vi "Test Turning Point.vi"() -> ()   [LabVIEW 2014]
uses:
  ZScan.ctl
panel:
  out "Z @ Max Sharpness":dbl
  out "Max Sharpness":sgl
  out "Waveform Chart":dbl(graph)
  out "XY Graph":cluster{"Displacements":dbl[], dbl[]}[](graph)
  in  "Focus Parameters":T1={"Z0"=3.0, "f0"=100.0, "curvature"=3.0, "noise"=2.0}
  in  "Z Scan Parameters":T2={"Z Range"=20.0, "Resolution"=1.0, "Initial Direction"=enum."Up", "Focus Threshold"=970.0, "Ascent Constant"=0.1} {"Focus Threshold" min=0.0 max=1000.0 step=1.0 format="%#_2f"; "Ascent Constant" min=0.0 max=1000.0 step=1.0 format="%#_2f"; "Resolution" min=0.0 max=1.0 step=0.01 format="%_2g"; "Z Range" format="%_3g"}
  # "LICENSED MATERIALS – PROPERTY OF IBM\nCopyright IBM Corp. 2016,\nALL RIGHTS RESERVED"
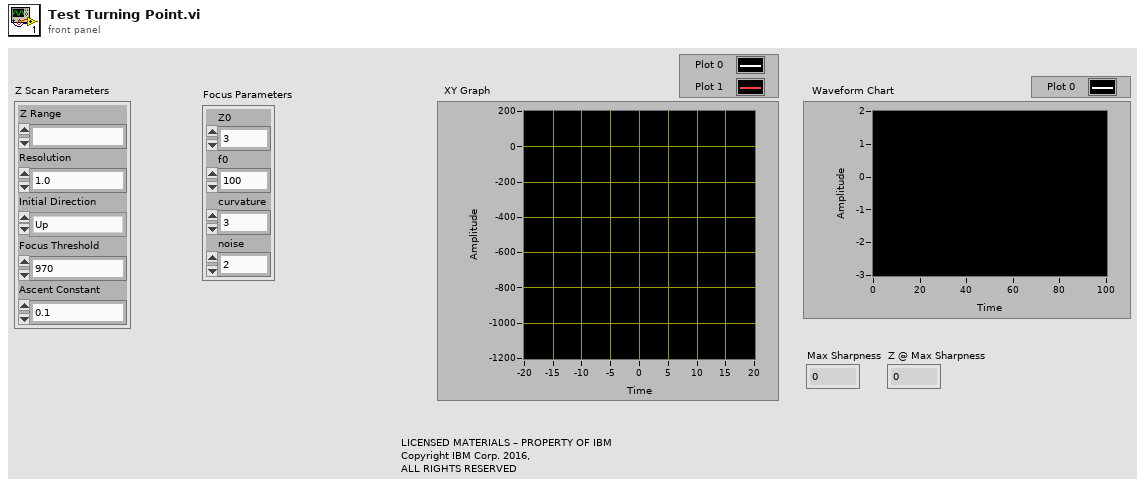
[diagram p1: front panel]
types:
  T1 = cluster{"Z0":dbl, "f0":dbl, "curvature":dbl, "noise":dbl}
  T2 = typedef "ZScan.ctl" = cluster{"Z Range":ext, "Resolution":dbl, "Initial Direction":enum16{"Up", "Down"}, "Focus Threshold":dbl, "Ascent Constant":dbl}
  T3 = cluster{"Registers Filled?":bool, "Negative Edge Slope?":bool, "Negative Z Slope?":bool, "Focus at Edge?":bool}
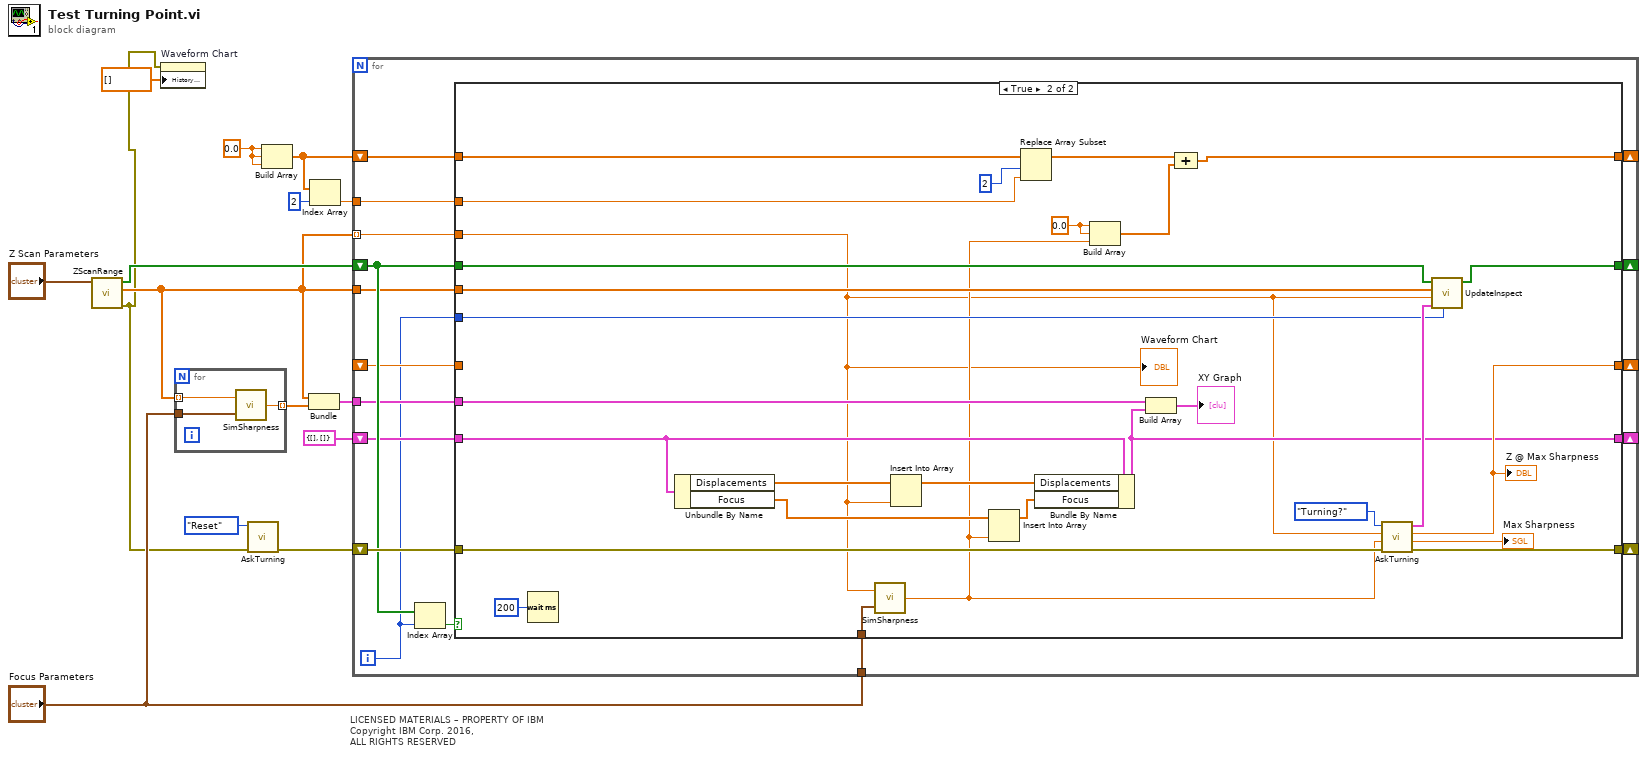
[diagram p0: block diagram]
diagram:
  w13 = 0.0 ("element")
  # "LICENSED MATERIALS – PROPERTY OF IBM\nCopyright IBM Corp. 2016,\nALL RIGHTS RESERVED"
  n1 = call "ZScanRange.vi"("Z Scan Parameters"="Z Scan Parameters") -> ("error out"=w1:errorcluster, "Displacements"=w5:dbl[], "Inspect?"=w8:bool[])  [unwired: 8 in]
  n2 = property on="Waveform Chart" class="WFChart (strict)"(error in=w1, "History Data"=dbl[] []) -> ()  [unwired: 1 in, 2 out]
  n3 = for {
    tunnel: "Focus Parameters" -> [w18]
    tunnel: [w17] -> w6 mode=indexing
    tunnel: w5 -> [w16] mode=indexing
    n4 = call "SimSharpness.vi"("Focus Parameters"=w18, "Z"=w16) -> ("Sharpness"=w17:dbl)
  }
  n5 = call "AskTurning.vi"("error in (no error)"=w1, "Function"=enum16{"Turning?", "Reset"}."Reset") -> ("error out"=w14:errorcluster)  [unwired: 6 in, 3 out]
  n6 = Build Array(w13, w13, w13) -> (w11:dbl[])
  n7 = Bundle("Displacements"=w5, w6) -> (w4:cluster{"Displacements":dbl[], dbl[]})  [unwired: 1 in]
  n8 = Index Array(array=w11, index=2) -> (element=w10:dbl)
  n9 = for {
    shift-right: [w33] -> _
    shift-left: w14 -> [w35]
    shift-right: [w32] -> _
    shift-left: w11 -> [w34]
    shift-right: [w31] -> _
    shift-left: w8 -> [w29]
    tunnel: w5 -> [w28]
    shift-right: [w27] -> _
    shift-left: _ -> [w26]
    tunnel: w5 -> [w24] mode=indexing
    tunnel: w10 -> [w25]
    tunnel: "Focus Parameters" -> [w23]
    tunnel: w4 -> [w22]
    shift-right: [w20] -> _
    shift-left: cluster{"Displacements":dbl[], "Focus":dbl[]} {"Displacements"=[], "Focus"=[]} -> [w21]
    i -> [w19]
    n10 = Index Array(array=w29, index=w19) -> (element=w30:bool)
    n11 = case shown="True" w30 {
      tunnel: w35 -> [w40 w55]
      tunnel: w34 -> [w39 w58]
      tunnel: [w40 w54] -> w33
      tunnel: [w39 w66] -> w32
      tunnel: w29 -> [w38 w65]
      tunnel: [w38 w64] -> w31
      tunnel: w28 -> [_ w63]
      tunnel: [w37 w62] -> w27
      tunnel: w26 -> [w37 _]
      tunnel: w19 -> [_ w60]
      tunnel: w25 -> [_ w59]
      tunnel: w24 -> [_ w42]
      tunnel: w23 -> [_ w53]
      tunnel: w22 -> [_ w51]
      tunnel: w21 -> [w36 w50]
      tunnel: [w36 w44] -> w20
      frame False {
      }
      frame True {
        w57 = 0.0 ("element")
        n12 = Wait (ms)(milliseconds to wait=u32 200) -> ()  [unwired: 1 out]
        n13 = Unbundle By Name(w50) -> ("Displacements"=w49:dbl[], "Focus"=w47:dbl[])
        n14 = call "SimSharpness.vi"("Focus Parameters"=w53, "Z"=w42) -> ("Sharpness"=w43:dbl)
        n15 = Insert Into Array(array=w49, new element=w42) -> (w48:dbl[])  [unwired: 1 in]
        n16 = Insert Into Array(array=w47, new element=w43) -> (w46:dbl[])  [unwired: 1 in]
        n17 = Replace Array Subset(array=w58, new element=w59, index=2) -> (w68:dbl[])
        n18 = Bundle By Name(cluster=w50, "Displacements"=w48, "Focus"=w46) -> (w44:cluster{"Displacements":dbl[], "Focus":dbl[]})
        n19 = Build Array(w57, w57, w43) -> (w56:dbl[])
        n20 = Build Array(w51, w44) -> (→"XY Graph":cluster{"Displacements":dbl[], "Focus":dbl[]}[])
        n21 = Compound Arithmetic op=ADD(w68, w56) -> (w66:dbl[])
        n22 = call "AskTurning.vi"("error in (no error)"=w55, "Edge Sherpness"=w43, "Z"=w42, "Function"=enum16{"Turning?", "Reset"}."Turning?") -> ("error out"=w54:errorcluster, "Max Sharpness"=→"Max Sharpness":sgl, "Z @ Max Sharpness"=w62:dbl, "Questions"=w61:T3)  [unwired: 4 in]
        "Z @ Max Sharpness" <- w62
        n23 = call "UpdateInspect.vi"("Current Id"=w60, "Answers"=w61, "Current Z"=w42, "Displacements"=w63, "Inspect? in"=w65) -> ("Inspect? out"=w64:bool[])  [unwired: 6 in]
        "Waveform Chart" <- w42
      }
    }
  }
